vi "Add Image.vi"(10 "Image Array In":i32[](array[numeric]), 11 "Pixel Array In":i32[](array[numeric])) -> (3 "Pixel Array Out":i32[](array[numeric]))   [LabVIEW 2018]
doc: "Overlays the white image array elements onto the pixel array, creating a fire 'source'."
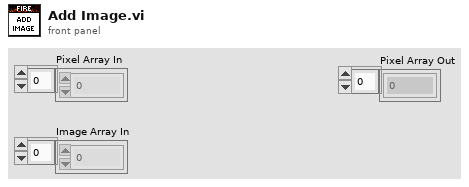
[diagram p1: front panel]
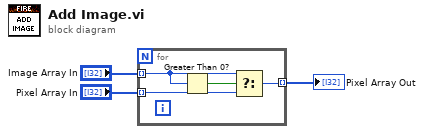
[diagram p0: block diagram]
diagram:
  n1 = for {
    tunnel: "Pixel Array In" -> [w4] mode=indexing
    tunnel: "Image Array In" -> [w5] mode=indexing
    tunnel: [w6] -> w1 mode=indexing
    n2 = Greater Than 0?(x=w5) -> (x > 0?=w7:bool)
    n3 = Select(t=w5, s=w7, f=w4) -> (s? t:f=w6:i32)
  }
  "Pixel Array Out" <- w1
